vi "Gen - Convert Int32 to String.vi"(11 "Num In":i32) -> (3 "String Out":string)   [LabVIEW 2020]
doc: "Convert string into Number in DBL format"
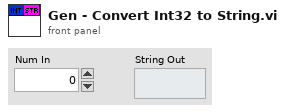
[diagram p1: front panel]
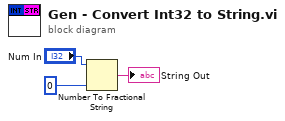
[diagram p0: block diagram]
diagram:
  n1 = Number To Fractional String(number="Num In", precision (6)=i16 0) -> (F-format string=→"String Out":string)  [unwired: 2 in]
